vi "Adv_Callback_Event.vi"(4 "LightField Automation in":refnum<class "LightField Automation.lvclass">, 5 "Event Data":cluster{"sender":refnum<k24>, "e":refnum<k24>}, 6 "Control Ref":refnum<k24>, 7 "Event Common Data":T1) -> ()   [LabVIEW 2015, in "LightField Automation.lvclass"]
uses:
  LightField Automation.lvclass
  C:/Program Files/Princeton Instruments/LightField/AddInViews/PrincetonInstruments.LightFieldViewV3.dll
  Program Files/Princeton Instruments/LightField/AddInViews/PrincetonInstruments.LightFieldViewV3.dll
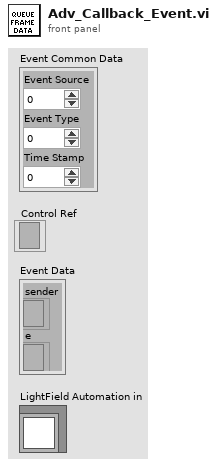
[diagram p1: front panel]
types:
  T1 = cluster{"Event Source":i32, "Event Type":u32, "Time Stamp":u32}
  T2 = cluster{"Image":dbl[][][], "Frame Size":cluster{"F":i32, "Y":i32, "X":i32}}[]
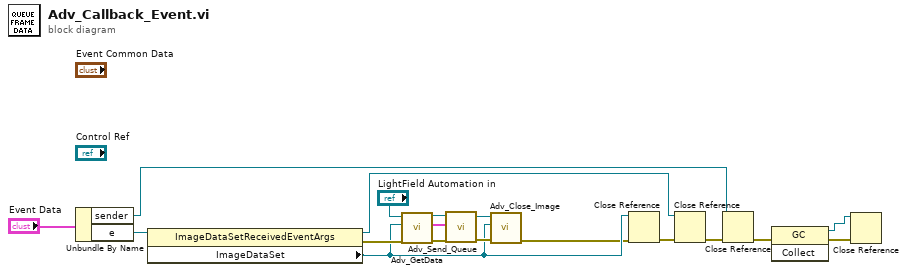
[diagram p0: block diagram]
diagram:
  n1 = Unbundle By Name("Event Data") -> ("sender"=w9:refnum<k24>, "e"=w13:refnum<k24>)
  n2 = property class="ImageDataSetReceivedEventArgs"(reference=w13) -> (reference out=w8:refnum<k24>, error out=w12:errorcluster, "ImageDataSet"=w2:refnum<k24>)  [unwired: 1 in]
  n3 = call "Adv_GetData.vi"("error in (no error)"=w12, "IImageDataSet"=w2, "LightField Automation in"="LightField Automation in") -> ("error out"=w17:errorcluster, "Data"=w16:T2, "LightField Automation out"=w15:refnum<class "LightField Automation.lvclass">)  [unwired: 6 in]
  n4 = call "Adv_Send_Queue.vi"("error in (no error)"=w17, "Data"=w16, "LightField Automation in"=w15) -> ("error out"=w4:errorcluster, "LightField Automation out"=w3:refnum<class "LightField Automation.lvclass">)  [unwired: 7 in]
  n5 = call "Adv_Close_Image.vi"("error in (no error)"=w4, "ImageDataSet"=w2, "LightField Automation in"=w3) -> ("error out"=w1:errorcluster)  [unwired: 7 in, 1 out]
  n6 = Close Reference(reference=w2, error in (no error)=w1) -> (error out=w11:errorcluster)
  n7 = Close Reference(reference=w8, error in (no error)=w11) -> (error out=w10:errorcluster)
  n8 = Close Reference(reference=w9, error in (no error)=w10) -> (error out=w7:errorcluster)
  n9 = invoke class="GC" method="Collect"(error in=w7) -> (reference out=w5:refnum<k24>, error out=w6:errorcluster)  [unwired: 2 in, 1 out]
  n10 = Close Reference(reference=w5, error in (no error)=w6) -> ()  [unwired: 1 out]
